vi "track_chunk.read.vi"(8 "error in":errorcluster, 10 "midi-file-events in":refnum<class "midi-file-events.lvclass">, 11 "midi-file in":refnum<class "midi-file.lvclass">) -> (0 "error out":errorcluster, 2 "midi-file-events out":refnum<class "midi-file-events.lvclass">, 3 "midi-file out":refnum<class "midi-file.lvclass">)   [LabVIEW 2020, in "midi-file.lvclass"]
uses:
  midi-file.lvclass
  midi-file-events/midi-file-events.lvclass
  midi-file.lvclass/midi-file.ctl
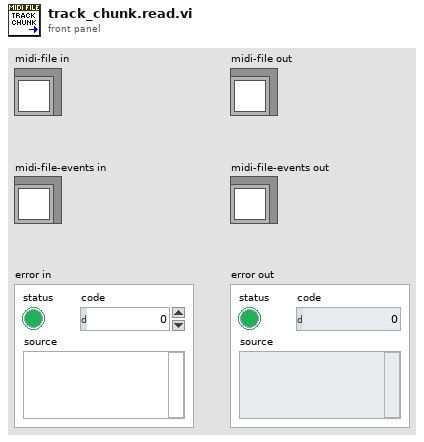
[diagram p1: front panel]
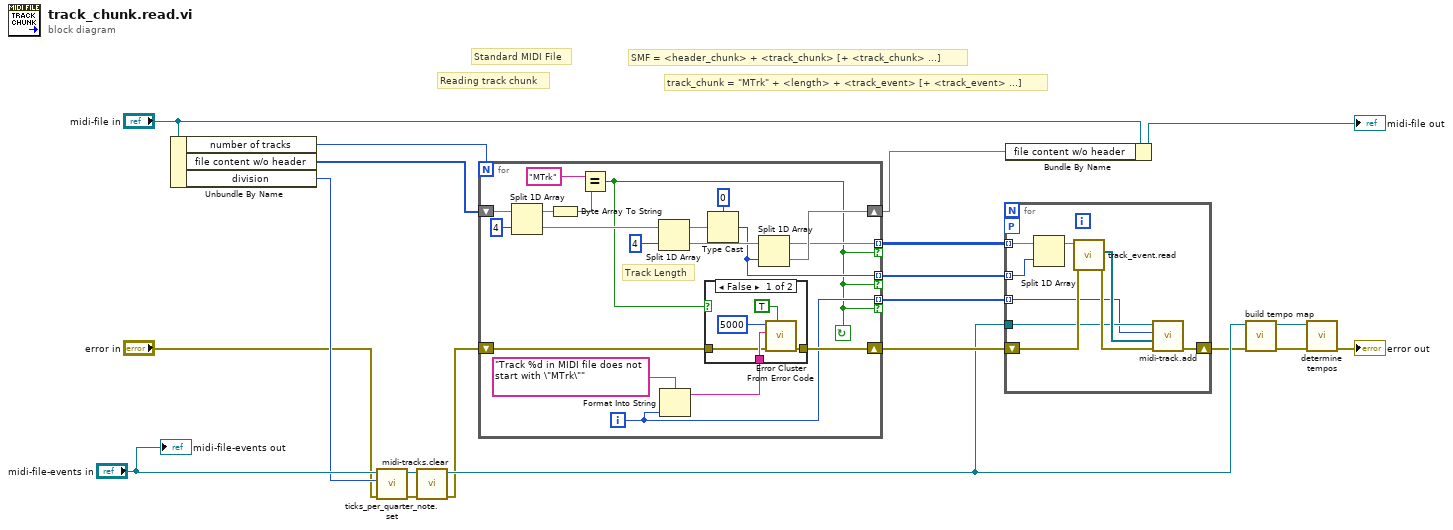
[diagram p0: block diagram]
diagram:
  # "track_chunk = \"MTrk\" + <length> + <track_event> [+ <track_event> ...]"
  # "Reading track chunk"
  # "Standard MIDI File"
  # "SMF = <header_chunk> + <track_chunk> [+ <track_chunk> ...]"
  n1 = Unbundle By Name("midi-file in") -> ("number of tracks"=w15:i16, "file content w/o header"=w18:u8[], "division"=w9:i16)
  n2 = call "ticks_per_quarter_note.set.vi"("error in (no error)"="error in", "ticks per quarter note (division)"=w9, "midi-file-events in"="midi-file-events in") -> ("error out"=w3:errorcluster, "midi-file-events out"=w11:refnum<class "midi-file-events.lvclass">)  [unwired: 7 in]
  n3 = call "midi-tracks.clear.vi"("error in (no error)"=w3, "midi-file-events in"=w11) -> ("error out"=w1:errorcluster, "midi-file-events out"=w7:refnum<class "midi-file-events.lvclass">)  [unwired: 8 in]
  n4 = for {
    N: w15 -> [_]
    shift-right: [w31] -> w14
    shift-left: w18 -> [w34]
    tunnel: [w30] -> w17 mode=indexing if=w21
    tunnel: [w29] -> w16 mode=indexing if=w21
    shift-right: [w24] -> w13
    shift-left: w1 -> [w23]
    tunnel: [w22] -> w12 mode=indexing if=w21
    i -> [w22]
    stop <- w21 continue-if-true
    # "Track Length"
    n5 = Split 1D Array(array=w34, index=4) -> (first subarray=w33:u8[], second subarray=w32:u8[])
    n6 = Byte Array To String(unsigned byte array=w33) -> (string=w28:string)
    n7 = Equal?(x="MTrk", y=w28) -> (x = y?=w21:bool)
    n8 = Split 1D Array(array=w32, index=4) -> (first subarray=w37:u8[], second subarray=w39:u8[])
    n9 = Format Into String(format string="Track %d in MIDI file does not start with \"MTrk\"" ("error message (\"\")"), w22) -> (resulting string=w25:string)  [unwired: 2 in, 1 out]
    n10 = case shown="False" w21 {
      tunnel: w25 -> [w43 _]
      tunnel: [w42 w45] -> w24
      tunnel: w23 -> [w41 w45]
      frame False {
        n11 = call <vilib>:"Error Cluster From Error Code.vi"("show call chain? (False)"=TRUE, "error in (no error)"=w41, "error message (\"\")"=w43, "error code (0)"=5000) -> ("error out"=w42:errorcluster)  [unwired: 5 in]
      }
      frame True {
      }
    }
    n12 = Type Cast(type=0, x=w37) -> (*(type *) &x=w29:i32)
    n13 = Split 1D Array(array=w39, index=w29) -> (first subarray=w30:u8[], second subarray=w31:u8[])
  }
  n14 = for {
    workers-P: _ -> [_]
    tunnel: w17 -> [w53] mode=indexing
    tunnel: w16 -> [w52] mode=indexing
    shift-right: [w48] -> w5
    shift-left: w13 -> [w51]
    tunnel: w7 -> [w47]
    tunnel: w12 -> [w46] mode=indexing
    n15 = Split 1D Array(array=w53, index=w52) -> (first subarray=w54:u8[])  [unwired: 1 out]
    n16 = call "track_event.read.vi"("error in"=w51, "Track Chunk Core"=w54) -> ("error out"=w49:errorcluster, "file events"=w50:refnum<class "midi-file-event.lvclass">[])  [unwired: 7 in, 1 out]
    n17 = call "midi-track.add.vi"("error in (no error)"=w49, "Track Events"=w50, "Track Number"=w46, "midi-file-events in"=w47) -> ("error out"=w48:errorcluster)  [unwired: 6 in, 1 out]
  }
  n18 = Bundle By Name(cluster="midi-file in", "file content w/o header"=w14) -> (→"midi-file out":refnum<class "midi-file.lvclass">)
  n19 = call "build tempo map.vi"("error in (no error)"=w5, "midi-file-events in"=w7) -> ("error out"=w4:errorcluster, "midi-file-events out"=w6:refnum<class "midi-file-events.lvclass">)  [unwired: 8 in]
  n20 = call "determine tempos.vi"("error in (no error)"=w4, "midi-file-events in"=w6) -> ("error out"=→"error out":errorcluster)  [unwired: 7 in, 2 out]
  "midi-file-events out" <- "midi-file-events in"
